vi "删除相同元素.vi"(0 "输入":cluster{"X":sgl, "Y":sgl}[](array[cluster])) -> (1 "输出":cluster{"X":sgl, "Y":sgl}[](array[cluster]), 2 "indices of removed elements":i32[](array[numeric]))   [LabVIEW 2018]
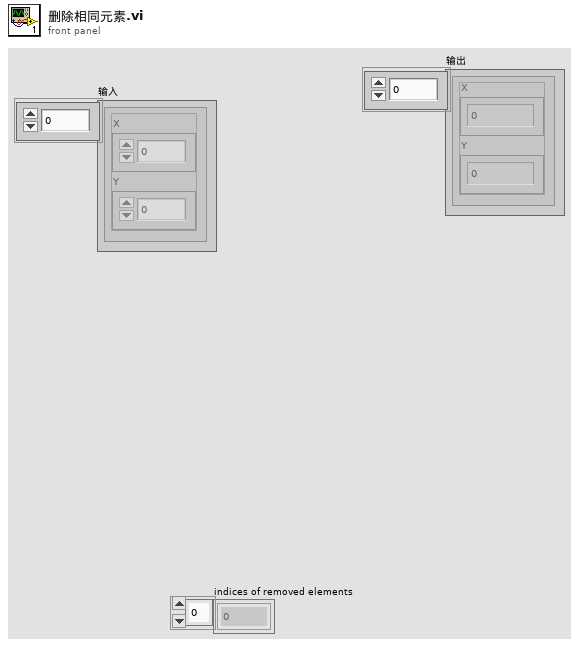
[diagram p1: front panel]
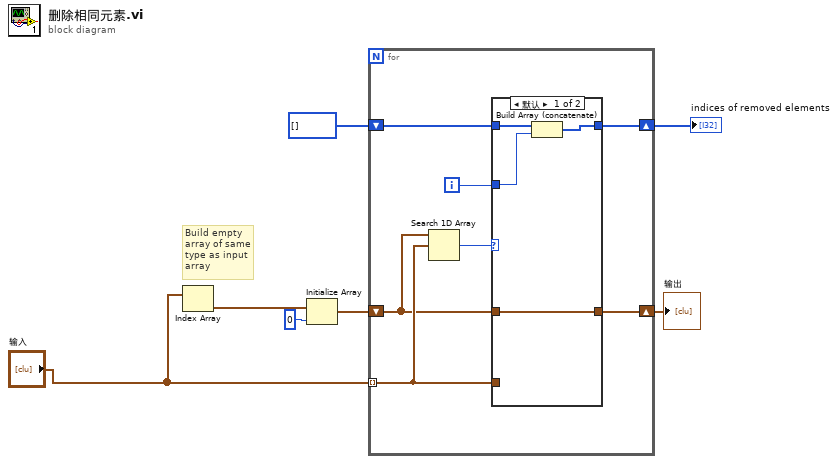
[diagram p0: block diagram]
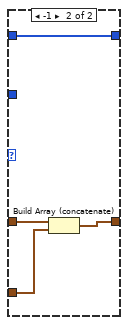
[diagram p2: hidden frame]
diagram:
  # "Build empty array of same type as input array"
  n1 = Index Array(array="输入") -> (element=w5:cluster{"X":sgl, "Y":sgl})  [unwired: 1 in]
  n2 = Initialize Array(w5, 0 ("Dimension Size")) -> (w4:cluster{"X":sgl, "Y":sgl}[])
  n3 = for {
    tunnel: "输入" -> [w13] mode=indexing
    shift-right: [w12] -> w1
    shift-left: w4 -> [w11]
    shift-right: [w9] -> w6
    shift-left: i32[] [] -> [w8]
    i -> [w10]
    n4 = Search 1D Array(1D array=w11, element=w13) -> (index of element=w14:i32)  [unwired: 1 in]
    n5 = case shown="默认" w14 {
      tunnel: w13 -> [_ w22]
      tunnel: [w18 w20] -> w12
      tunnel: w11 -> [w18 w21]
      tunnel: w10 -> [w15 _]
      tunnel: [w16 w19] -> w9
      tunnel: w8 -> [w17 w19]
      frame Default {
        n6 = Build Array (concatenate)(w17, w15) -> (w16:i32[])
      }
      frame -1 {
        n7 = Build Array (concatenate)(w21, w22) -> (w20:cluster{"X":sgl, "Y":sgl}[])
      }
    }
  }
  "indices of removed elements" <- w6
  "输出" <- w1
